vi "blink.vi"() -> ()   [LabVIEW 2010]
panel:
  in  "stop":bool
  out "Boolean":bool
  # "Page 1"
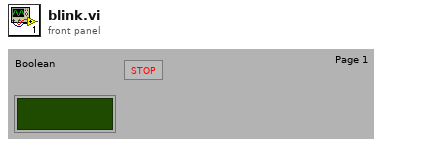
[diagram p1: front panel]
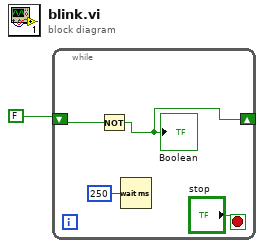
[diagram p0: block diagram]
diagram:
  n1 = while {
    shift-right: [w3] -> _
    shift-left: FALSE ("Boolean") -> [w4]
    stop <- "stop" stop-if-true
    n2 = Not(x=w4) -> (.not. x?=w3:bool)
    "Boolean" <- w3
    n3 = Wait (ms)(milliseconds to wait=u32 250) -> ()  [unwired: 1 out]
  }
